vi "Initialise ctrl values.vi"(8 "error in (no error)":errorcluster) -> (0 "error out":errorcluster)   [LabVIEW 2017]
uses:
  Typedefs/HW config states enum.ctl
  Typedefs/Read Write Enum.ctl
  Typedefs/AOL modes.ctl
  Global Variables/gl_UI Ctrl Refs.vi
  Global Variables/General Globals.vi
  Typedefs/Laser control knob.ctl
  Typedefs/PMT control knob.ctl
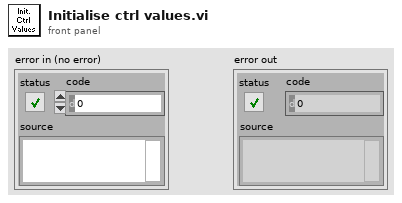
[diagram p1: front panel]
types:
  T1 = typedef "HW config states enum.ctl" = enum16{"Load from file", "Save to file", "Write all", "Read all", "Write XY stage settings", "Write DAQ FPGA settings", "Write Control FPGA settings", "Write Phys Channels", "Write System Config", "Write HW Config", "Save System Config", "Save HW Config", "Clear", "Compare from file"}
  T2 = typedef "UI ctrl refs cluster.ctl" = cluster{"Top level VI path":path, "Top level VI ref":refnum<vi>, "User menu ref":refnum<k9>, "Sub Panel control":refnum<vi>, "Imaging Param Tab":refnum<vi>, "Occurrence-Start drivers":refnum<k4>, "Occurrence-Speed logging initialised":refnum<k4>, "Occurrence-XYZ stage initialised":refnum<k4>, "Exit button":refnum<vi>, "Status ind":refnum<vi>, "Set as origin":refnum<vi>, "Speed Logging":refnum<vi>, "Time Lapse":refnum<vi>, "Live Imaging":refnum<vi>, "AOL Z Stack":refnum<vi>, "Motor Z Stack":refnum<vi>, "Funct Acq button":refnum<vi>, "Hard Shutter":refnum<vi>, "Virtual Shutter":refnum<vi>, "Laser Power":refnum<vi>, "AOL Mode":refnum<vi>, "Frame Size":refnum<vi>, "Field of View":refnum<vi>, "Dwell Time":refnum<vi>, "Zoom":refnum<vi>, "AOL Z":refnum<vi>, "Objective":refnum<vi>, "Axis":refnum<vi>, "Paths & Names":refnum<vi>, "Experiment folder path (ind.)":refnum<vi>, "Last State (Ind.)":refnum<vi>, "Averages":refnum<vi>, "Angle (degrees)":refnum<vi>, "X centre":refnum<vi>, "Y centre":refnum<vi>, "Plane Mode":refnum<vi>, "# Planes":refnum<vi>, "Z Start":refnum<vi>, "Z Stop":refnum<vi>, "Z Step":refnum<vi>, "PMT 1":refnum<vi>, "PMT 2":refnum<vi>, "Stage XYZ Position":refnum<vi>, "Pockels@Z Start":refnum<vi>, "Pockels@Z Stop":refnum<vi>, "Obtain Z Start":refnum<vi>, "Obtain Z Stop":refnum<vi>, "Live stim.trig.period":refnum<vi>, "Live stim.trig.enable":refnum<vi>, "XY Stage Move":refnum<vi>, "Funct. Acq. Pockels Modulation":refnum<vi>, "Enable Video Recording":refnum<vi>, "Video Record-Live Imaging":refnum<vi>, "Video Record-Funct acq":refnum<vi>, "AOL Z-stack Chirps Ready (ind)":refnum<vi>, "Center freq ind (nm)":refnum<vi>, "Pickup mode (ind)":refnum<vi>, "Logging queue (ind)":refnum<vi>, "Back aperture power (ind.)":refnum<vi>, "Power after objective (ind.)":refnum<vi>, "Switch user":refnum<vi>, "Ls1 Conn. Status":refnum<vi>, "Ls1Tuning Status":refnum<vi>, "Ls1 Faults":refnum<vi>, "Ls1 Connection":refnum<vi>, "Ls1 Mode":refnum<vi>, "Ls1 POWER [mW]":refnum<vi>, "Ls1Shutter":refnum<vi>, "Ls1 Wavelength":refnum<vi>, "Ls1 Note":refnum<vi>, "Ls1 Confirm Wav":refnum<vi>, "Ls1 PreChrp Prism1":refnum<vi>, "Ls1 PreChrp Prism2":refnum<vi>, "Ls1 wav top Ind":refnum<vi>, "Ls1 power top Ind":refnum<vi>, "Ls1 Pump peak Hold":refnum<vi>, "Ls1 Status Ind":refnum<vi>, "Ls1 wav cancel":refnum<vi>, "Experiment Type":refnum<vi>, "Biology Information":refnum<vi>}
  T3 = typedef "System Configuration.ctl" = cluster{"Laser wavelength (nm)":dbl, "DAQ FPGA System":T4, "Control system":T5}
  T4 = typedef "DAQ FPGA system config.ctl" = cluster{"Clock Freq (MHz) ":dbl, "Samples Wait after Trigger":u16, "AOD fill":u16, "StartupDelay":i32, "Slip Cycle (clock cycles)":u32, "Add Cycle":bool}
  T5 = typedef "CTRL system config.ctl" = cluster{"AOD 1 Amplitude":i16, "AOD 2 Amplitude":i16, "AOD 3 Amplitude":i16, "AOD 4 Amplitude":i16, "AOD 5 Amplitude":i16, "AOD 6 Amplitude":i16, "T0 (ns)":dbl, "Ta (ns)":dbl, "Data Time Interval (ns)":dbl, "Ctrl FPGA Clock (MHz)":dbl}
  T6 = typedef "AOL_Globals.ctl" = cluster{"Imaging Protocol":T7, "Number of POI":u16, "Number of Miniscans":u16, "Number of Trials":u16, "Number of Cycles ":u64, "# Averaged Frames":u16, "Laser power (%)":u8, "Pockels (V)":dbl, "Acquisition Length (sec)":dbl, "Fill time (us)":dbl, "POI Dwell time (us)":dbl, "Miniscan Dwell time per pixel (us)":dbl, "PMT 1":dbl, "PMT 2":dbl, "Back Apperture (mA)":dbl, "Frame Size":T8, "Center Frequency":dbl, "Field of View (norm)":dbl, "DwellTime (us)":dbl, "Wavelength (nm)":dbl, "Zoom":dbl, "AOL Z":dbl, "AOL Mode":T9, "GridXY":dbl, "GridZ":dbl, "TriggerPeriod (sec)":dbl, "Number of Pixels in Miniscan":u16, "Experiment folder path":path, "X centre":dbl, "Y centre":dbl, "Angle (degrees)":dbl, "Plane Mode":T10, "Threshold":u16[], "Regenerate Chirps":bool, "Rectangle ROI length (pixels)":u16, "Rectangle ROI height (pixels)":u16, "AOD fill":u16, "StartupDelay":i32, "Samples Wait after Trigger":u16, "Slip Cycle":u32, "Add Cycle":bool, "Functional Mode":T11, "Z Start":dbl, "Z Stop":dbl, "# Planes":i32}
  T7 = typedef "Imaging Protocols enum.ctl" = enum16{"AOL Z-Stack", "Motor Z Stack", "Functional Acquisition", "Single Plane Acquisition", "Volume Acquisition", "Live Imaging", "Live Plane Imaging", "Live Volume Imaging"}
  T8 = typedef "Frame Size.ctl" = u16
  T9 = typedef "AOL modes.ctl" = enum16{"Raster", "Structural", "Pointing", "Mini Scan", "Alignment"}
  T10 = typedef "Plane Mode.ctl" = u16
  T11 = typedef "Functional Mode.ctl" = enum16{"Point", "Line", "Patch", "Plane", "Volume"}
  T12 = enum8{"Enabled", "Disabled", "Disabled and Grayed Out"}
  T13 = typedef "Laser control knob.ctl" = u16
  T14 = typedef "Read Write Enum.ctl" = enum16{"Read", "Write"}
  T15 = typedef "PMT control knob.ctl" = u16
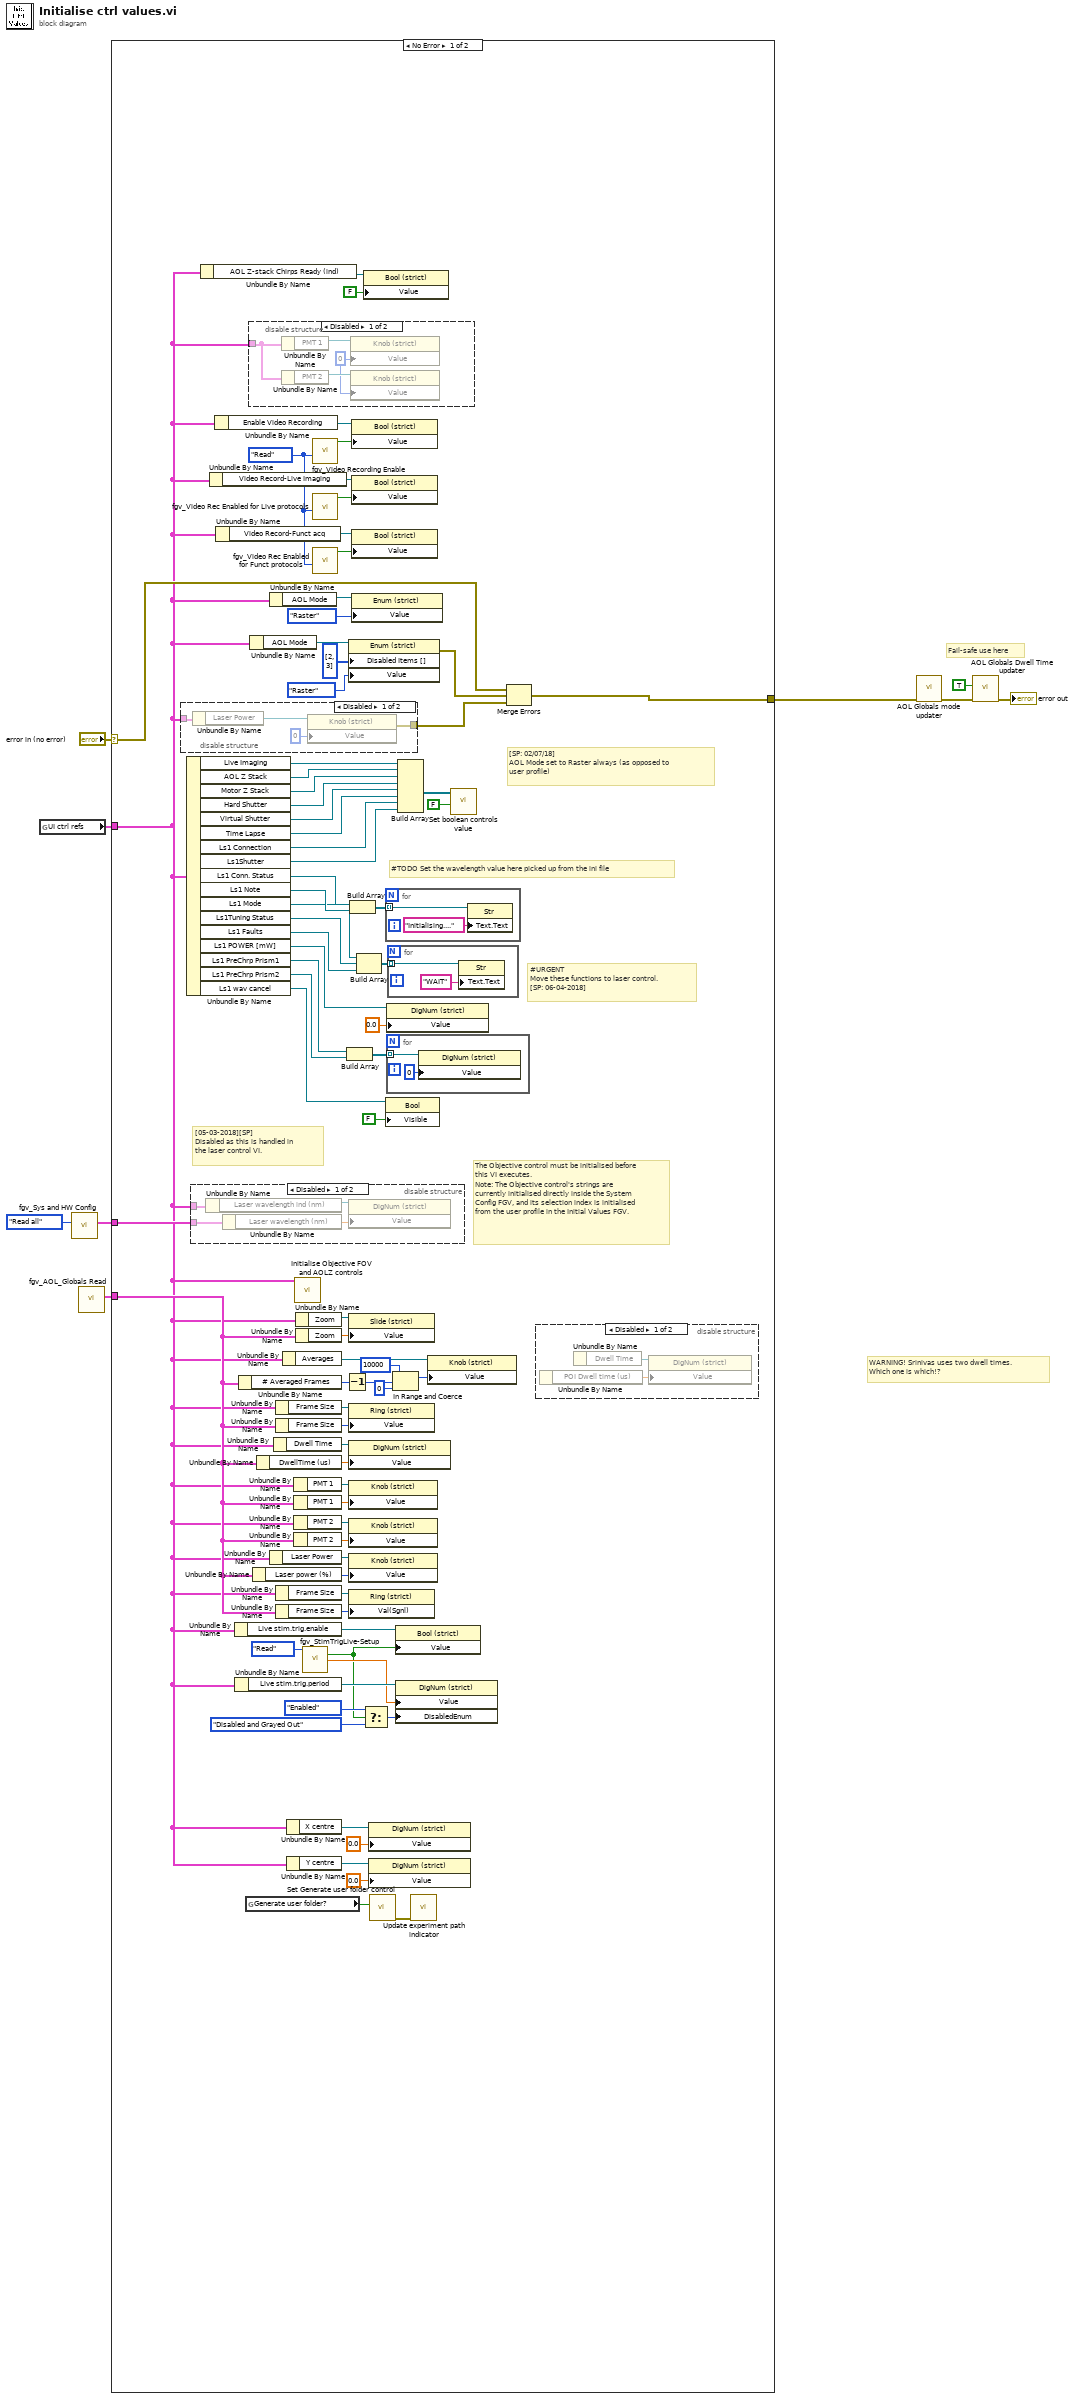
[diagram p0: block diagram]
diagram:
  # "Fail-safe use here"
  # "WARNING! Srinivas uses two dwell times.\nWhich one is which!?"
  n1 = global read "gl_UI Ctrl Refs.vi" "UI ctrl refs"() -> (w8:T2)
  n2 = call "fgv_Sys and HW Config.vi"("Function"=HW_config_states_enum."Read all") -> ("System Config OUT"=w1:T3)  [unwired: 8 in, 2 out]
  n3 = call "fgv_AOL_Globals Read.vi"() -> ("AOL_Globals"=w6:T6)  [unwired: 9 in, 2 out]
  n4 = case shown="No Error" "error in (no error)" {
    selector: "error in (no error)" -> [w31 w109]
    tunnel: w8 -> [w10 _]
    tunnel: [w76 w109] -> w5
    tunnel: w6 -> [w11 _]
    tunnel: w1 -> [w37 _]
    frame No Error {
      w71 = Read_Write_Enum."Read" ("Function")
      # "[SP: 02/07/18]\nAOL Mode set to Raster always (as opposed to \nuser profile)"
      # "#URGENT \nMove these functions to laser control.\n[SP: 06-04-2018]"
      # "[05-03-2018][SP]\nDisabled as this is handled in \nthe laser control VI."
      # "#TODO Set the wavelength value here picked up from the ini file"
      # "The Objective control must be initialised before this VI executes.\nNote: The Objective control's strings are currently initialised directly inside the System Config FGV, and its selection index is initialised from the user profile in the Initial Values FGV."
      n5 = disable-structure shown="Disabled" {
        disable-tunnel: [w102 _] -> w77
        disable-tunnel: w10 -> [w101 _]
        frame Disabled {
          n6 = Unbundle By Name(w101) -> ("Laser Power"=w104:refnum<vi>)
          n7 = property class="Knob (strict)"(reference=w104, "Value"=T13 0) -> (error out=w102:errorcluster)  [unwired: 1 in, 1 out]
        }
        frame Enabled {
        }
      }
      n8 = Unbundle By Name(w10) -> ("Live Imaging"=w88:refnum<vi>, "AOL Z Stack"=w87:refnum<vi>, "Motor Z Stack"=w86:refnum<vi>, "Hard Shutter"=w85:refnum<vi>, "Virtual Shutter"=w84:refnum<vi>, "Time Lapse"=w81:refnum<vi>, "Ls1 Connection"=w29:refnum<vi>, "Ls1Shutter"=w28:refnum<vi>, "Ls1 Conn. Status"=w27:refnum<vi>, "Ls1 Note"=w26:refnum<vi>, "Ls1 Mode"=w23:refnum<vi>, "Ls1Tuning Status"=w22:refnum<vi>, "Ls1 Faults"=w21:refnum<vi>, "Ls1 POWER [mW]"=w20:refnum<vi>, "Ls1 PreChrp Prism1"=w18:refnum<vi>, "Ls1 PreChrp Prism2"=w17:refnum<vi>, "Ls1 wav cancel"=w15:refnum<vi>)
      n9 = disable-structure shown="Disabled" {
        disable-tunnel: w37 -> [w90 _]
        disable-tunnel: w10 -> [w89 _]
        frame Disabled {
          n10 = Unbundle By Name(w89) -> ("Laser wavelength ind (nm)"=w92:refnum<vi>)
          n11 = Unbundle By Name(w90) -> ("Laser wavelength (nm)"=w91:dbl)
          n12 = property on="Property Node" class="DigNum (strict)"(reference=w92, "Value"=w91) -> ()  [unwired: 1 in, 2 out]
        }
        frame Enabled {
        }
      }
      n13 = Unbundle By Name(w10) -> ("AOL Z-stack Chirps Ready (ind)"=w65:refnum<vi>)
      n14 = Unbundle By Name(w10) -> ("Video Record-Live Imaging"=w70:refnum<vi>)
      n15 = Unbundle By Name(w10) -> ("Enable Video Recording"=w73:refnum<vi>)
      n16 = Unbundle By Name(w10) -> ("Video Record-Funct acq"=w69:refnum<vi>)
      n17 = Unbundle By Name(w10) -> ("Live stim.trig.enable"=w44:refnum<vi>)
      n18 = Unbundle By Name(w10) -> ("Live stim.trig.period"=w43:refnum<vi>)
      n19 = Unbundle By Name(w11) -> ("# Averaged Frames"=w61:u16)
      n20 = global read "General Globals.vi" "Generate user folder?"() -> (w30:bool)
      n21 = disable-structure shown="Disabled" {
        disable-tunnel: w10 -> [w106 _]
        frame Disabled {
          w105 = T15 0 ("Value")
          n22 = Unbundle By Name(w106) -> ("PMT 1"=w108:refnum<vi>)
          n23 = Unbundle By Name(w106) -> ("PMT 2"=w107:refnum<vi>)
          n24 = property on="Property Node" class="Knob (strict)"(reference=w108, "Value"=w105) -> ()  [unwired: 1 in, 2 out]
          n25 = property on="Property Node" class="Knob (strict)"(reference=w107, "Value"=w105) -> ()  [unwired: 1 in, 2 out]
        }
        frame Enabled {
        }
      }
      n26 = Unbundle By Name(w10) -> ("AOL Mode"=w79:refnum<vi>)
      n27 = Unbundle By Name(w11) -> ("Laser power (%)"=w46:u8)
      n28 = Unbundle By Name(w11) -> ("DwellTime (us)"=w52:dbl)
      n29 = Unbundle By Name(w10) -> ("AOL Mode"=w75:refnum<vi>)
      n30 = Unbundle By Name(w10) -> ("Laser Power"=w47:refnum<vi>)
      n31 = Unbundle By Name(w10) -> ("Dwell Time"=w53:refnum<vi>)
      n32 = Unbundle By Name(w10) -> ("Frame Size"=w54:refnum<vi>)
      n33 = Unbundle By Name(w11) -> ("Frame Size"=w55:T8)
      n34 = Unbundle By Name(w10) -> ("Frame Size"=w66:refnum<vi>)
      n35 = Unbundle By Name(w11) -> ("Frame Size"=w45:T8)
      n36 = Unbundle By Name(w10) -> ("Averages"=w60:refnum<vi>)
      n37 = Unbundle By Name(w10) -> ("X centre"=w36:refnum<vi>)
      n38 = Unbundle By Name(w10) -> ("Y centre"=w35:refnum<vi>)
      n39 = Unbundle By Name(w10) -> ("PMT 1"=w50:refnum<vi>)
      n40 = Unbundle By Name(w11) -> ("PMT 1"=w49:dbl)
      n41 = Unbundle By Name(w10) -> ("PMT 2"=w51:refnum<vi>)
      n42 = Unbundle By Name(w11) -> ("PMT 2"=w48:dbl)
      n43 = call "Initialise Objective FOV and AOLZ controls.vi"("UI ctrl refs"=w10) -> ()  [unwired: 10 in, 1 out]
      n44 = Unbundle By Name(w10) -> ("Zoom"=w63:refnum<vi>)
      n45 = Unbundle By Name(w11) -> ("Zoom"=w62:dbl)
      n46 = call "fgv_StimTrigLive-Setup.vi"("Function"=enum16{"Intialize", "Write", "Read", "Clear"}."Read") -> ("Live stim.trig.enable"=w32:bool, "Live stim.trig.period (sec)"=w41:dbl)  [unwired: 11 in, 2 out]
      n47 = call "fgv_Video Recording Enable.vi"("Function"=w71) -> ("Video Recording Enabled"=w72:bool)  [unwired: 10 in]
      n48 = call "fgv_Video Rec Enabled for Live protocols.vi"("Function"=w71) -> ("Video Recording Enabled for Live protocols"=w67:bool)  [unwired: 10 in]
      n49 = call "fgv_Video Rec Enabled for Funct protocols.vi"("Function"=w71) -> ("Video Recording Enabled for functional acq protocols"=w68:bool)  [unwired: 10 in]
      n50 = Decrement(x=w61) -> (x-1=w59:u16)
      n51 = Build Array(w18, w17) -> (w16:refnum<vi>[])
      n52 = property on="Property Node" class="Enum (strict)"(reference=w79, "Disabled Items []"=i32[] [2, 3], "Value"=AOL_modes."Raster") -> (error out=w78:errorcluster)  [unwired: 1 in, 1 out]
      n53 = property on="Property Node" class="Slide (strict)"(reference=w63, "Value"=w62) -> ()  [unwired: 1 in, 2 out]
      n54 = property on="Property Node" class="Ring (strict)"(reference=w54, "Value"=w55) -> ()  [unwired: 1 in, 2 out]
      n55 = property on="Property Node" class="DigNum (strict)"(reference=w53, "Value"=w52) -> ()  [unwired: 1 in, 2 out]
      n56 = property class="Knob (strict)"(reference=w50, "Value"=w49) -> ()  [unwired: 1 in, 2 out]
      n57 = property class="Knob (strict)"(reference=w51, "Value"=w48) -> ()  [unwired: 1 in, 2 out]
      n58 = property class="Knob (strict)"(reference=w47, "Value"=w46) -> ()  [unwired: 1 in, 2 out]
      n59 = property on="Property Node" class="Ring (strict)"(reference=w66, "Val(Sgnl)"=w45) -> ()  [unwired: 1 in, 2 out]
      n60 = Build Array(w27, w26) -> (w25:refnum<vi>[])
      n61 = property on="Property Node" class="Bool (strict)"(reference=w73, "Value"=w72) -> ()  [unwired: 1 in, 2 out]
      n62 = property on="Property Node" class="Bool (strict)"(reference=w70, "Value"=w67) -> ()  [unwired: 1 in, 2 out]
      n63 = property on="Property Node" class="Bool (strict)"(reference=w69, "Value"=w68) -> ()  [unwired: 1 in, 2 out]
      n64 = property on="Property Node" class="Enum (strict)"(reference=w75, "Value"=AOL_modes."Raster") -> ()  [unwired: 1 in, 2 out]
      n65 = Build Array(w23, w22, w21) -> (w24:refnum<vi>[])
      n66 = property class="Bool (strict)"(reference=w65, "Value"=FALSE) -> ()  [unwired: 1 in, 2 out]
      n67 = Select(t=T12."Enabled" ("Disabled"), s=w32, f=T12."Disabled and Grayed Out" ("Disabled")) -> (s? t:f=w40:T12)
      n68 = property class="DigNum (strict)"(reference=w36, "Value"=0.0) -> ()  [unwired: 1 in, 2 out]
      n69 = property class="DigNum (strict)"(reference=w35, "Value"=0.0) -> ()  [unwired: 1 in, 2 out]
      n70 = call "Set Generate user folder control.vi"("Generate user folder?"=w30) -> ("error out"=w12:errorcluster)  [unwired: 10 in]
      n71 = for {
        tunnel: w25 -> [w98] mode=indexing
        n72 = property class="Str"(reference=w98, "Text.Text"="Initialising....") -> ()  [unwired: 1 in, 2 out]
      }
      n73 = property class="Bool"(reference=w15, "Visible"=FALSE) -> ()  [unwired: 1 in, 2 out]
      n74 = property class="DigNum (strict)"(reference=w20, "Value"=0.0) -> ()  [unwired: 1 in, 2 out]
      n75 = for {
        tunnel: w16 -> [w94] mode=indexing
        n76 = property class="DigNum (strict)"(reference=w94, "Value"=0) -> ()  [unwired: 1 in, 2 out]
      }
      n77 = for {
        tunnel: w24 -> [w96] mode=indexing
        n78 = property class="Str"(reference=w96, "Text.Text"="WAIT") -> ()  [unwired: 1 in, 2 out]
      }
      n79 = In Range and Coerce(upper limit=u16 10000, x=w59, lower limit=u16 0) -> (coerced(x)=w58:u16)  [unwired: 1 out]
      n80 = property on="Property Node" class="Bool (strict)"(reference=w44, "Value"=w32) -> ()  [unwired: 1 in, 2 out]
      n81 = property on="Property Node" class="DigNum (strict)"(reference=w43, "Value"=w41, "DisabledEnum"=w40) -> ()  [unwired: 1 in, 2 out]
      n82 = Build Array(w88, w87, w86, w85, w84, w81, w29, w28) -> (w83:refnum<vi>[])
      n83 = call "Update experiment path indicator.vi"("error in (no error)"=w12) -> ()  [unwired: 9 in, 2 out]
      n84 = property on="Property Node" class="Knob (strict)"(reference=w60, "Value"=w58) -> ()  [unwired: 1 in, 2 out]
      n85 = call "Set boolean controls value.vi"("Value"=FALSE, "Boolean ctrl ref array"=w83) -> ()  [unwired: 10 in]
      n86 = Merge Errors(w31, w78, w77) -> (w76:errorcluster)
      n87 = disable-structure shown="Disabled" {
        frame Disabled {
          n88 = Unbundle By Name() -> ("POI Dwell time (us)"=w100:dbl)  [unwired: 1 in]
          n89 = Unbundle By Name() -> ("Dwell Time"=w99:refnum<vi>)  [unwired: 1 in]
          n90 = property on="Property Node" class="DigNum (strict)"(reference=w99, "Value"=w100) -> ()  [unwired: 1 in, 2 out]
        }
        frame Enabled {
        }
      }
    }
    frame Error {
    }
  }
  n91 = call "AOL Globals mode updater.vi"("error in"=w5) -> ("error out"=w4:errorcluster)  [unwired: 10 in]
  n92 = call "AOL Globals Dwell Time updater.vi"("error in"=w4, "Disable message (F)"=TRUE) -> ("error out"=→"error out":errorcluster)  [unwired: 9 in]
